vi "2MotorFinalKinematics.vi"() -> ()   [LabVIEW 2017]
uses:
  <vilib>/Platform/TimedLoop/XDataNode/timing_clust.ctl
  <vilib>/Platform/TimedLoop/XDataNode/nitl_modes.ctl
  <vilib>/Platform/TimedLoop/XDataNode/wakeup.ctl
  <vilib>/platform/TimedLoop/XDataNode/XDataNode.xnode
  <vilib>/Platform/TimedLoop/XDataNode/XDNodeRunTimeDep.lvlib
  <vilib>/Analysis/NI_AALPro.lvlib
panel:
  out "Numeric":dbl
  in  "Q1 decreases (right)":dbl
  in  "Q1 increases (left)":dbl
  in  "Kd 2":dbl(slide) scale=0.0..0.5
  in  "Ki 2":dbl(slide) scale=0.0..10.0
  in  "Kp 2":dbl(slide) scale=0.01..50.0
  in  "Manual\nControl":bool
  in  "X 2":dbl
  in  "Y 2":dbl
  out "Q1 (Bottom Motor)":dbl
  out "Q2":dbl
  in  "stop":bool
  out "Bottom motor":cluster{"Numeric":dbl, "Ref 2":dbl}(graph)
  out "top motor":cluster{"Numeric":dbl, "Ref 1":dbl}(graph)
  out "Analog 2":dbl(knob) scale=0.0..5.0
  out "Analog 1":dbl(knob) scale=0.0..5.0
  out "Pos 2":dbl(knob) scale=0.0..360.0
  out "Pos 1":dbl(knob) scale=0.0..360.0
  in  "Initialize Int 2":bool
  in  "Initialize Int 1":bool
  in  "Q 2":dbl(slide) scale=-180.0..180.0
  in  "Q 1":dbl(slide) scale=-180.0..180.0
  in  "Kd":dbl(slide) scale=0.0..0.5
  in  "Ki":dbl(slide) scale=0.0..10.0
  in  "Kp":dbl(slide) scale=0.01..50.0
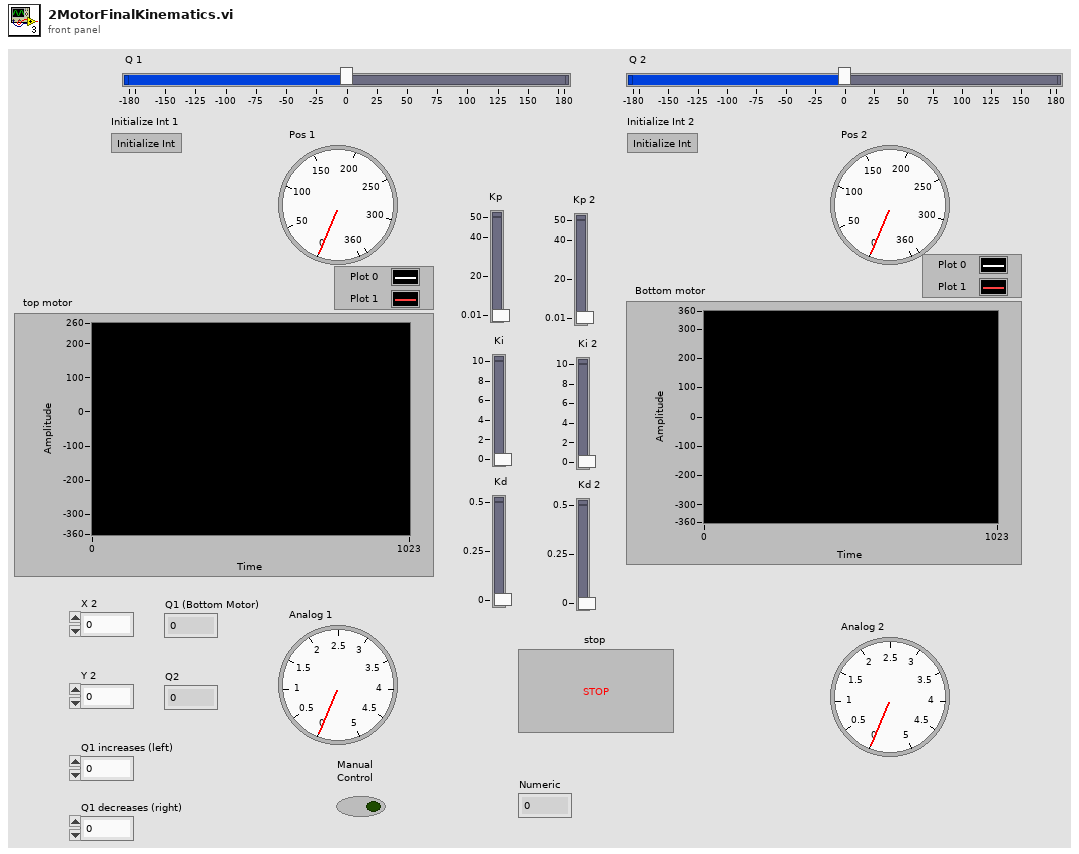
[diagram p1: front panel]
types:
  T1 = typedef "XDNodeRunTimeDep.lvlib/timing_clust.ctl" = cluster{"Expected End [f-1]":u64, "Actual End [f-1]":u64, "Finished Late? [f-1]":bool, "Expected End [i-1]":u64, "Actual End [i-1]":u64, "Finished Late? [i-1]":bool, "Expected Start [i]":u64, "Actual Start [i]":u64, "Expected Start [f]":u64, "Actual Start [f]":u64, "Source Name":string, "Structure Name":string, "Period":i64, "Deadline":i64, "Offset":i64, "Start":i64, "Priority":i32, "Timeout":i32, "Mode":T2, "Wakeup Reason":T3, "Error":errorcluster, "Source Type":string, "Secondary Source Type":string, "Global End Time":u64, "Global Start Time":u64, "Frame Duration":u64, "Iteration Duration":u64, "Assigned CPU":i32, "I/O Scan Engine Mode":u32}
  T2 = typedef "XDNodeRunTimeDep.lvlib/nitl_modes.ctl" = enum32{"No Change", "Process missed periods, maintain original phase", "Discard missed periods, maintain original phase", "Process missed periods, ignore original phase", "Discard missed periods, ignore original phase"}
  T3 = typedef "XDNodeRunTimeDep.lvlib/wakeup.ctl" = enum32{"Normal", "Aborted", "Asynchronous wakeup", "Timing source error", "Timed loop error", "Timeout"}
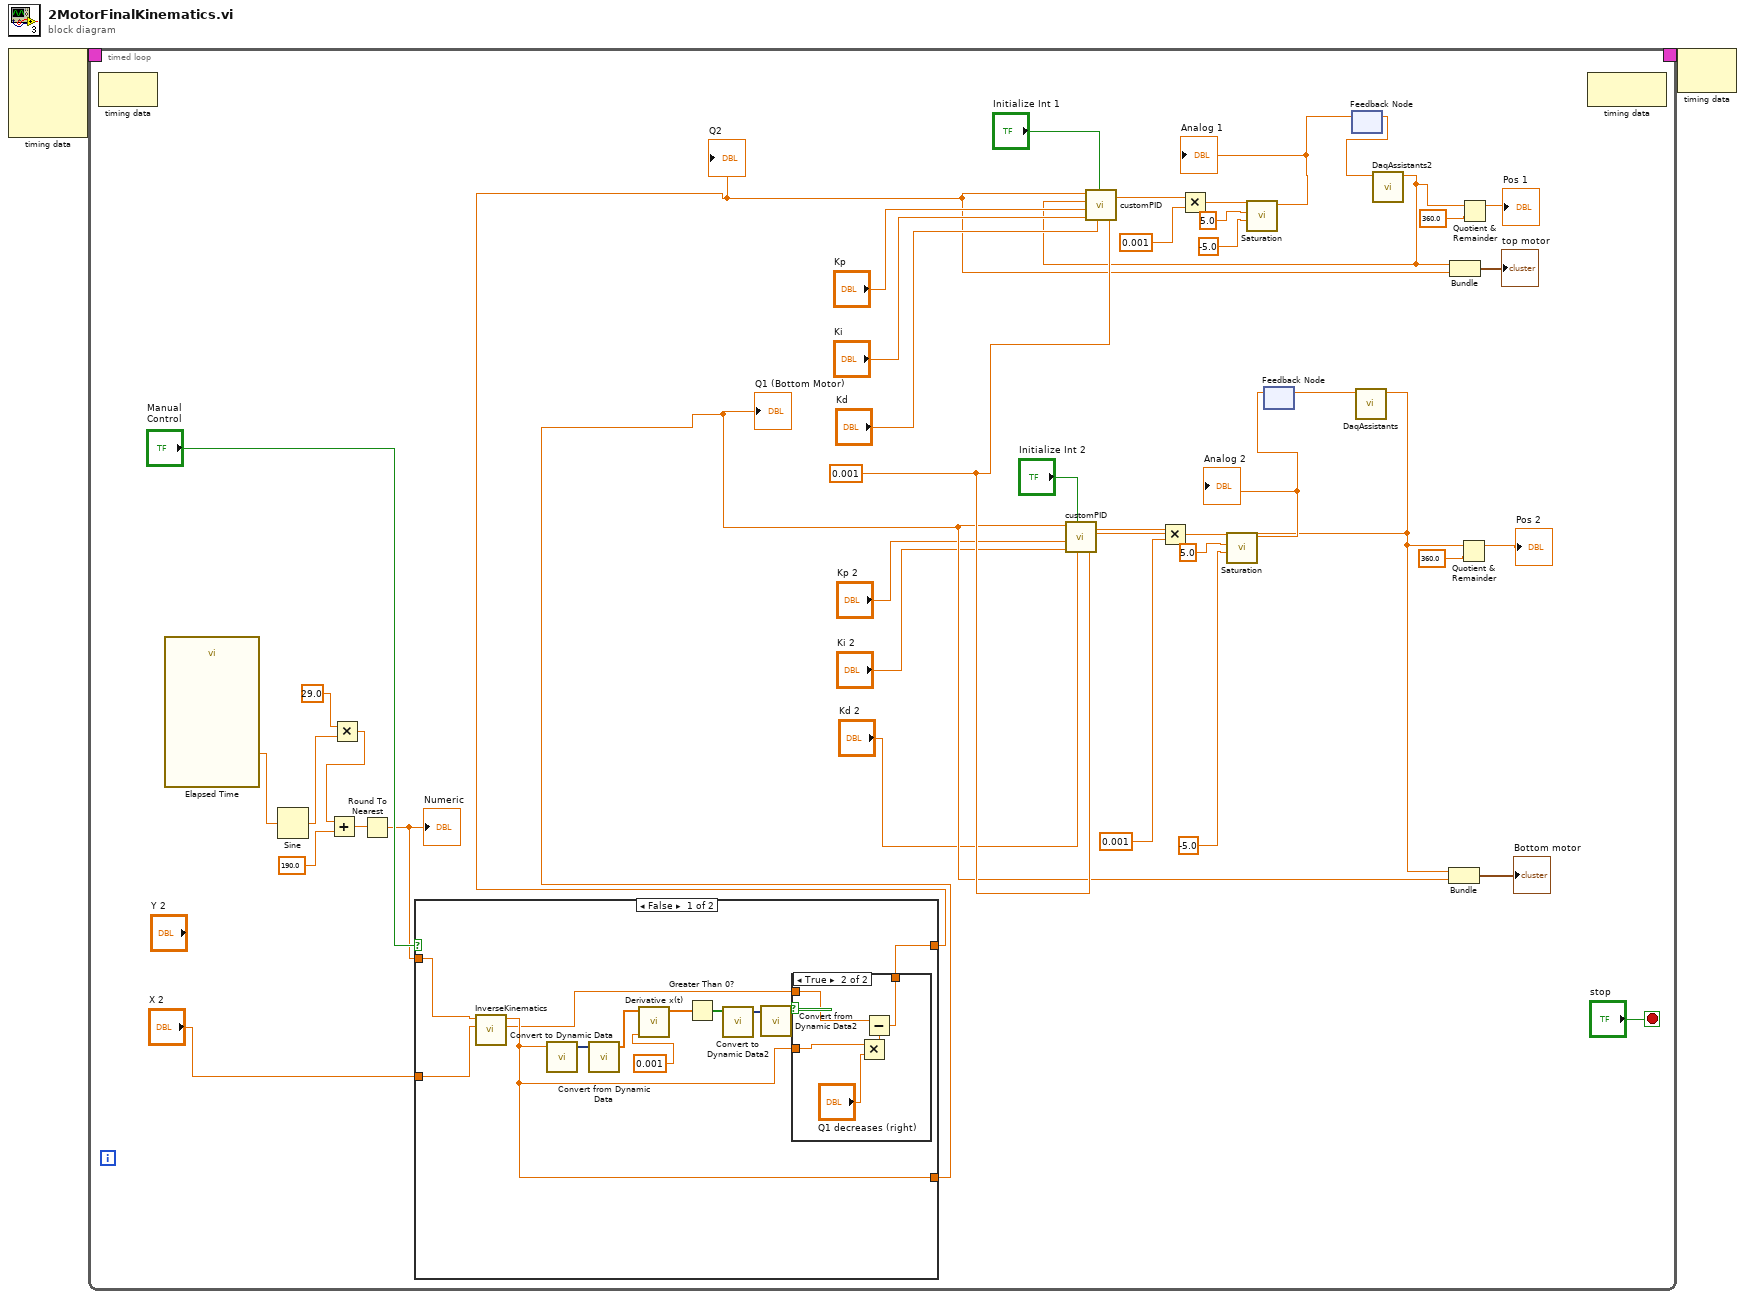
[diagram p0: block diagram]
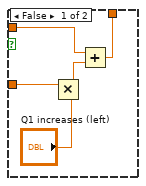
[diagram p2: hidden frame]
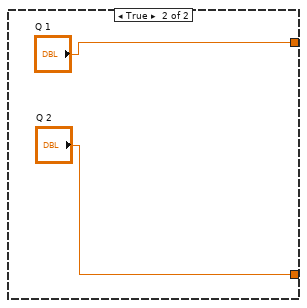
[diagram p3: hidden frame]
diagram:
  n1 = node-c288() -> (w2:T1)  [unwired: 4 in]
  n2 = timed-loop {
    timing: w2 -> [_]
    timing-out: [_] -> w1
    stop <- "stop" stop-if-true
    w23 = 0.001
    n3 = node-c288() -> ()  [unwired: 1 in, 1 out]
    n4 = call "Elapsed Time"() -> ("Elapsed Time (s)"=w9:dbl)  [unwired: 12 in, 7 out]
    n5 = Sine(x=w9) -> (sin(x)=w6:dbl)
    n6 = Multiply(x=29.0, y=w6) -> (x*y=w5:dbl)
    n7 = Add(x=w5, y=190.0) -> (x+y=w4:dbl)
    n8 = Round To Nearest(number=w4) -> (nearest integer value=w3:dbl)
    "Numeric" <- w3
    n9 = case shown="False" "Manual\nControl" {
      tunnel: [w47 "Q 1"] -> w19
      tunnel: [w48 "Q 2"] -> w18
      tunnel: w3 -> [w57 _]
      tunnel: "X 2" -> [w56 _]
      frame False {
        n10 = call "InverseKinematics.vi"("X"=w56, "Y"=w57) -> ("Q2"=w46:dbl, "Q1"=w48:dbl)  [unwired: 8 in]
        n11 = call "Convert to Dynamic Data"("Double"=w48) -> ("Dynamic Data Type"=w54:dynamicdata)  [unwired: 3 in]
        n12 = call "Convert from Dynamic Data"("Dynamic Data Type"=w54) -> ("Array"=w53:dbl[])  [unwired: 3 in]
        n13 = call <vilib>:"Derivative x(t).vi"("dt"=0.001, "X"=w53) -> ("dX/dt"=w55:dbl[])  [unwired: 8 in, 1 out]
        n14 = Greater Than 0?(x=w55) -> (x > 0?=w50:bool[])
        n15 = call "Convert to Dynamic Data2"("Array"=w50) -> ("Dynamic Data Type"=w49:dynamicdata)  [unwired: 3 in]
        n16 = call "Convert from Dynamic Data2"("Dynamic Data Type"=w49) -> ("Scalar"=w51:bool)  [unwired: 3 in]
        n17 = case shown="True" w51 {
          tunnel: w48 -> [w62 w66]
          tunnel: w46 -> [w60 w64]
          tunnel: [w59 w67] -> w47
          frame False {
            n18 = Multiply(x=w62, y="Q1 increases (left)") -> (x*y=w61:dbl)
            n19 = Add(x=w60, y=w61) -> (x+y=w59:dbl)
          }
          frame True {
            n20 = Multiply(x=w66, y="Q1 decreases (right)") -> (x*y=w65:dbl)
            n21 = Subtract(x=w64, y=w65) -> (x-y=w67:dbl)
          }
        }
      }
      frame True {
      }
    }
    "Q2" <- w19
    "Q1 (Bottom Motor)" <- w18
    n22 = feedback #1() -> (w11:dbl)  [unwired: 1 in]
    n23 = feedback #2() -> (w13:dbl)  [unwired: 1 in]
    n24 = call "DaqAssistants.vi"("output"=w11) -> ("Numeric"=w10:dbl)  [unwired: 10 in]
    n25 = call "customPID.vi"("dt"=w23, "Kd"="Kd 2", "Initialize"="Initialize Int 2", "Ki"="Ki 2", "Kp"="Kp 2", "Measured"=w10, "Desired"=w18) -> ("Motor Input"=w33:dbl)
    n26 = Multiply(x=w33, y=0.001) -> (x*y=w32:dbl)
    n27 = call "Saturation.vi"("lower bound"=-5.0, "upper bound"=5.0, "input"=w32) -> ("output"=w22:dbl)  [unwired: 8 in]
    "Analog 2" <- w22
    n28 = feedback-in #1(w22) -> ()
    n29 = call "DaqAssistants2.vi"("output"=w13) -> ("Numeric"=w12:dbl)  [unwired: 10 in]
    n30 = call "customPID.vi"("dt"=w23, "Kd"="Kd", "Initialize"="Initialize Int 1", "Ki"="Ki", "Kp"="Kp", "Measured"=w12, "Desired"=w19) -> ("Motor Input"=w44:dbl)
    n31 = Multiply(x=w44, y=0.001) -> (x*y=w43:dbl)
    n32 = call "Saturation.vi"("lower bound"=-5.0, "upper bound"=5.0, "input"=w43) -> ("output"=w21:dbl)  [unwired: 8 in]
    "Analog 1" <- w21
    n33 = feedback-in #2(w21) -> ()
    n34 = Bundle("Numeric"=w10, "Q 2"=w18) -> (→"Bottom motor":cluster{"Numeric":dbl, "Q 2":dbl})  [unwired: 1 in]
    n35 = Bundle("Numeric"=w12, "Q 1"=w19) -> (→"top motor":cluster{"Numeric":dbl, "Q 1":dbl})  [unwired: 1 in]
    n36 = Quotient & Remainder(x=w10, y=360.0) -> (x-y*floor(x/y)=→"Pos 2":dbl)  [unwired: 1 out]
    n37 = Quotient & Remainder(x=w12, y=360.0) -> (x-y*floor(x/y)=→"Pos 1":dbl)  [unwired: 1 out]
    n38 = node-c288() -> ()  [unwired: 1 in, 1 out]
  }
  n39 = node-c288(w1) -> ()  [unwired: 1 out]
